vi "Write Positions.vi"(8 "error in (no error)":errorcluster, 10 "Positions":i32[](array[numeric]), 11 "Focus Class in":refnum<class "Focus Class.lvclass">) -> (0 "error out":errorcluster, 3 "Focus Class out":refnum<class "Focus Class.lvclass">)   [LabVIEW 2024, in "Focus Class.lvclass"]
uses:
  Focus Class.lvclass
  Focus Class.lvclass/Focus Class.ctl
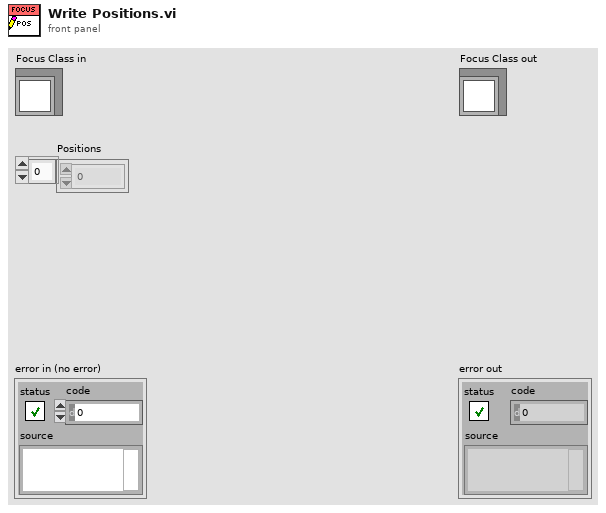
[diagram p1: front panel]
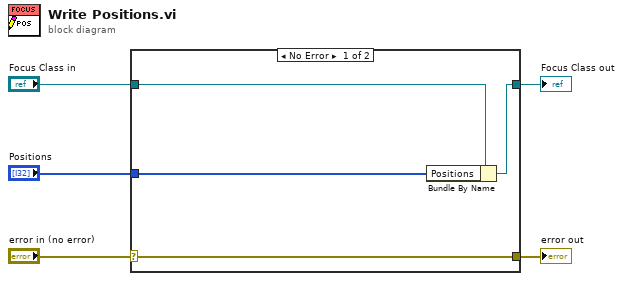
[diagram p0: block diagram]
diagram:
  n1 = case shown="No Error" "error in (no error)" {
    selector: "error in (no error)" -> [w9 w10]
    tunnel: [w9 w10] -> w4
    tunnel: [w7 w11] -> w2
    tunnel: "Focus Class in" -> [w8 w11]
    tunnel: "Positions" -> [w6 _]
    frame No Error {
      n2 = Bundle By Name(cluster=w8, "Positions"=w6) -> (w7:refnum<class "Focus Class.lvclass">)
    }
    frame Error {
    }
  }
  "error out" <- w4
  "Focus Class out" <- w2
